vi "Add Data to EQE Log File.vi"(4 "Skip cell?":bool, 6 "Scan settings":T1={"J-V scan"=TRUE, "J-t scan"=FALSE, "Min voltage (V)"=0.0, "Max voltage (V)"=1.4, "Step (V)"=0.01, "Measurement delay (ms)"=10.0, "1st scan FB-SC"=TRUE, "Inverted structure"=FALSE, "Stabilisation time (s)"=0.0, "Stabilisation mode"=0, "Stabilisation value (V or A) "=0.0, "Step time (s)"=1.0, "Integration time"=0, "Repeat light scans"=FALSE, "Stabilisation in the dark?"=FALSE, "J-t Min (V)"=0.0, "J-t Max (V)"=1.4, "J-t Step (V)"=0.01, "Max. power stabilisation"=FALSE, "J-t 1st scan FB-SC"=TRUE, "J-t Inverted structure"=FALSE, "Max power tracking"=FALSE, "Vmp (V)"=0.7, "Total stabilisation time (s)"=100.0, "J-t best pixel only"=0, "Max power best pixel only"=0, "Vmp from J-V scan"=FALSE, "Intensity dependence"=FALSE, "P dep best pixel only"=0, "External quantum efficiency"=FALSE, "EQE best pixel only"=0, "WL min (nm)"=300.0, "WL max (nm)"=900.0, "WL step (nm)"=5.0, "Wait (ms)"=100.0, "No. of repeat scans"=2.0, "Only repeat for best pixel"=0, "Chopper Freq.  (Hz)"=90.0, "Time Constant (s)"=2.0, "Stabilisation time step (s)"=1.0, "Illumination conditions"=2, "Scan rate min (V/s)"=0.1, "Scan rate max (V/s)"=1.0, "No. of scan rate steps"=1.0, "Scan rate voltage step priority"=FALSE, "Scan rate measurement delay priority"=FALSE, "J-t Illumination conditions"=0, "White bias  (no. of suns)"=200.0, "Max P stab. Specific voltage"=FALSE} {"J-t Illumination conditions" items=["Light only", "Dark only", "Light then dark", "Dark then light"]; "No. of scan rate steps" min=1.0 step=1.0; "Illumination conditions" items=["Light only", "Dark only", "Light then dark", "Dark then light", "Light then dark then light", "Dark then light then dark"]; "Time Constant (s)" items=["0.003", "0.01", "0.03", "0.1", "0.3", "1", "3", "10", "30", "100"]; "Only repeat for best pixel" items=["only for best pixel", "for best 2 pixels", "for best 3 pixels", "for best 4 pixels", "for best 5 pixels", "for best 6 pixels", "for best 7 pixels", "for all pixels"]; "No. of repeat scans" min=1.0 step=1.0; "EQE best pixel only" items=["only the best pixel", "the best 2 pixel", "the best 3 pixel", "the best 4 pixel", "the best 5 pixel", "the best 6 pixel", "the best 7 pixel", "all pixels"]; "P dep best pixel only" items=["only the best pixel", "the best 2 pixels", "the best 3 pixels", "the best 4 pixels", "the best 5 pixels", "the best 6 pixels", "the best 7 pixels", "all pixels"]; "Max power best pixel only" items=["only the best pixel", "the best 2 pixels", "the best 3 pixels", "the best 4 pixels", "the best 5 pixels", "the best 6 pixels", "the best 7 pixels", "all pixels"]; "J-t best pixel only" items=["only the best pixel", "the best 2 pixels", "the best 3 pixels", "the best 4 pixels", "the best 5 pixels", "the best 6 pixels", "the best 7 pixels", "all pixels"]; "Integration time" items=["Fast", "Normal", "High Accuracy"]; "Stabilisation mode" items=["V", "I"]; "Measurement delay (ms)" min=10.0}, 7 "Cell details cluster":T3={"Cell Position"=16, "Cell Label"="", "Pixel to measure"=0, "Area (cm^2)"=0.126, "Variable"="", "Variable value"="", "Scan settings in queue"=0, "Light or dark"="", "Measurement Type"=""} {"Pixel to measure" items=["All", "1", "2", "3", "4", "5", "6", "7", "8"]}, 8 "EQE Data Output Folder":path, 9 "Mismatch Factor":dbl, 10 "Jsc @ 1 sun (mA/cm^2)":dbl, 11 "File path for EQE data":path) -> (0 "File path for EQE image":path, 1 "EQE Curve":cluster{"all rows":dbl[], "all rows":dbl[]}[](graph) caption="JV Curve", 2 "File path for master log":path, 3 "Master Log":string[][](table))   [LabVIEW 2011]
uses:
  TypeDefs/Scan settings.ctl
  TypeDefs/Settings Boolean.ctl
  <vilib>/Utility/file.llb/Read From Spreadsheet File (DBL).vi
  <vilib>/Utility/file.llb/Write To Spreadsheet File (string).vi
  <vilib>/Utility/file.llb/Read From Spreadsheet File (string).vi
panel:
  in  "Experiment title":string
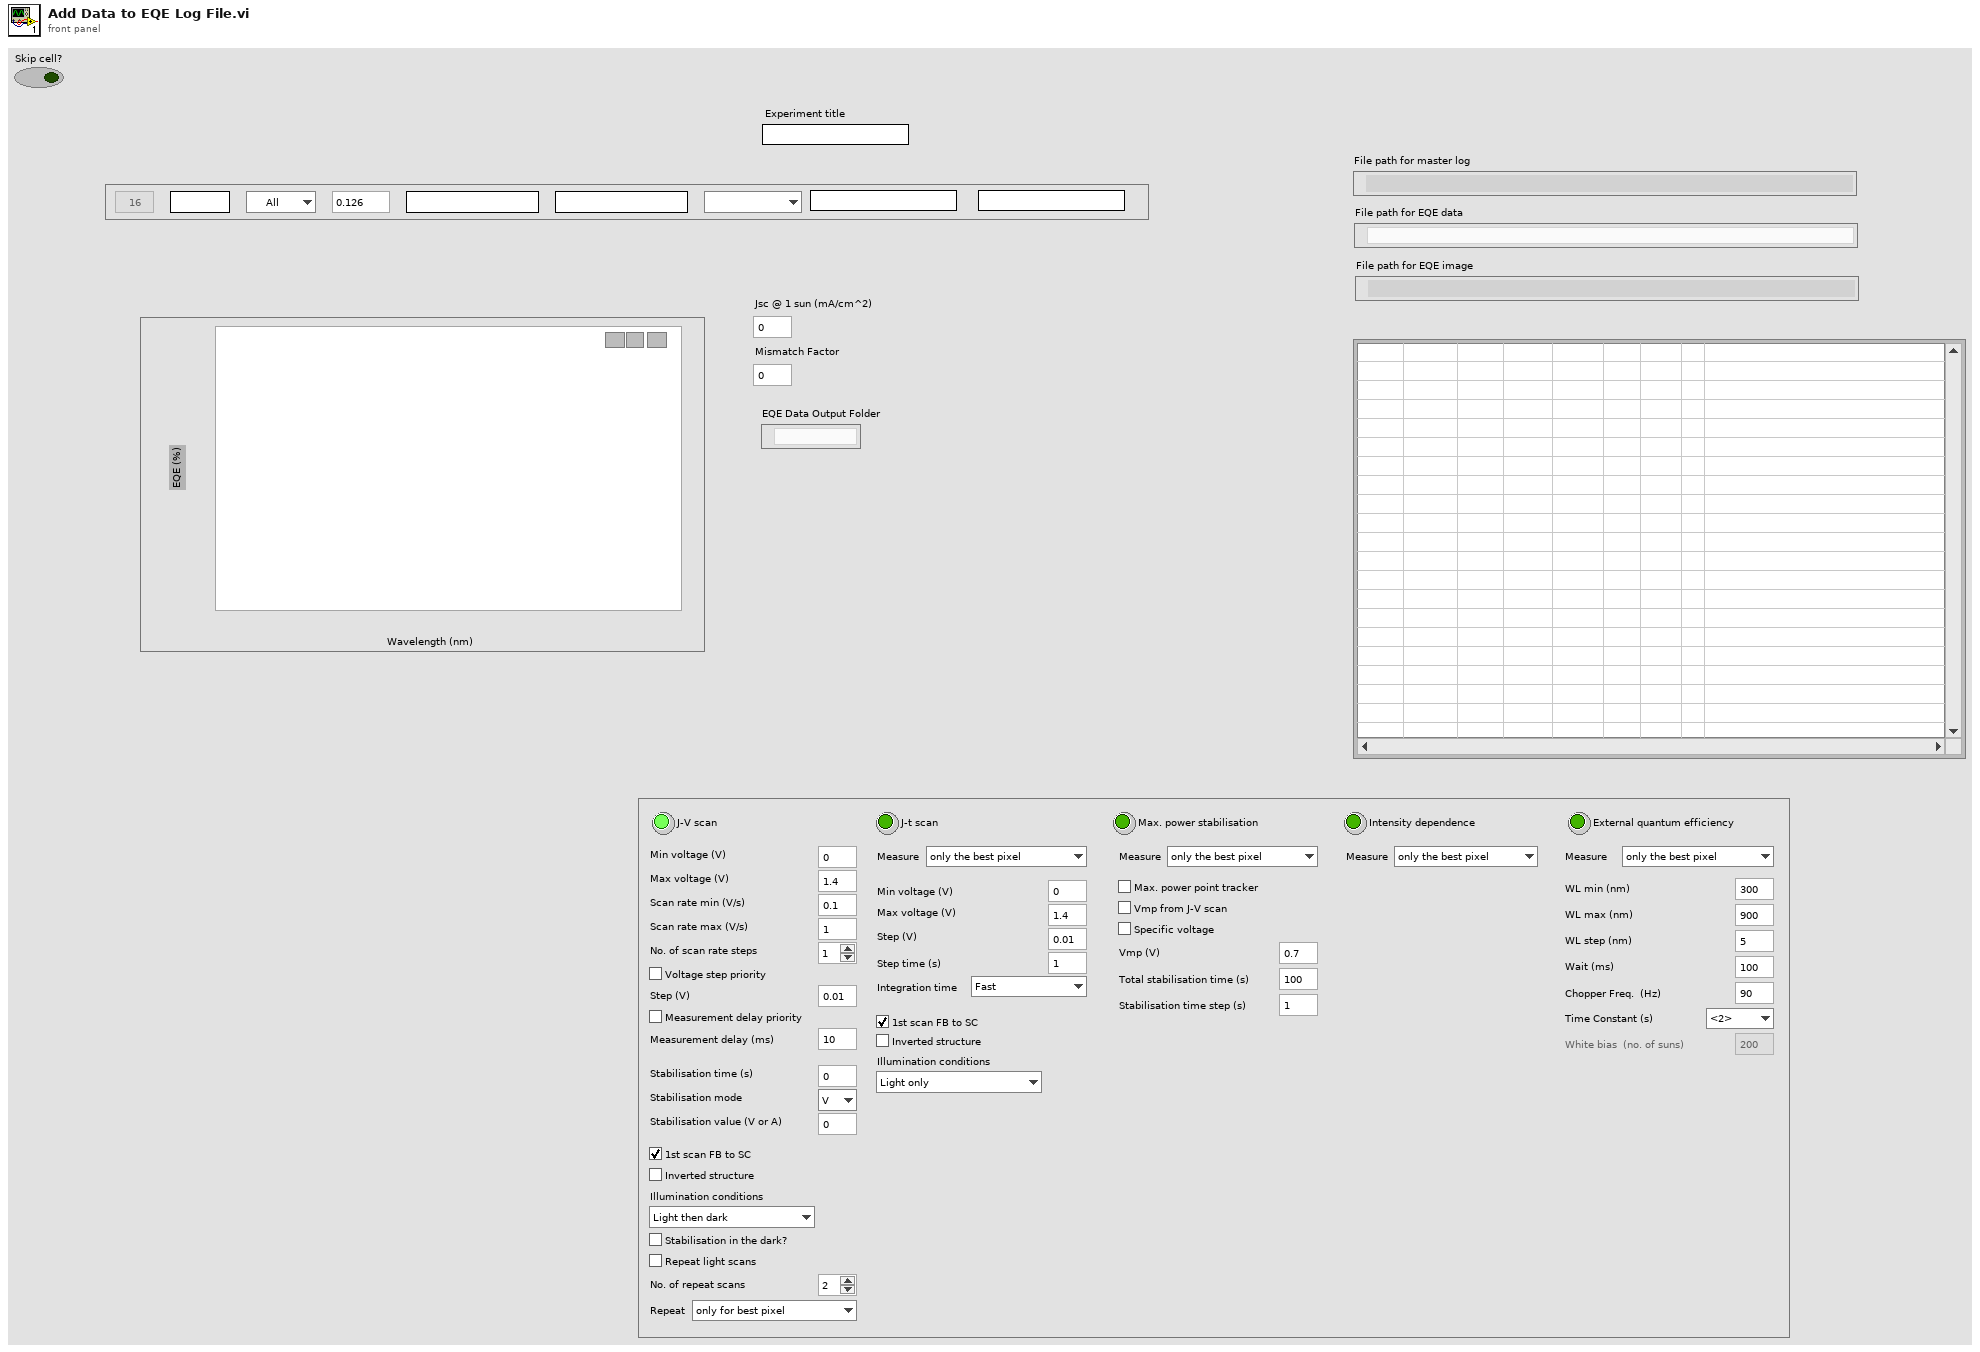
[diagram p1: front panel]
types:
  T1 = typedef "Scan settings.ctl" = cluster{"J-V scan":T2, "J-t scan":bool, "Min voltage (V)":dbl, "Max voltage (V)":dbl, "Step (V)":dbl, "Measurement delay (ms)":dbl, "1st scan FB-SC":bool, "Inverted structure":bool, "Stabilisation time (s)":dbl, "Stabilisation mode":u16, "Stabilisation value (V or A) ":dbl, "Step time (s)":dbl, "Integration time":u16, "Repeat light scans":bool, "Stabilisation in the dark?":bool, "J-t Min (V)":dbl, "J-t Max (V)":dbl, "J-t Step (V)":dbl, "Max. power stabilisation":bool, "J-t 1st scan FB-SC":bool, "J-t Inverted structure":bool, "Max power tracking":bool, "Vmp (V)":dbl, "Total stabilisation time (s)":dbl, "J-t best pixel only":u16, "Max power best pixel only":u16, "Vmp from J-V scan":bool, "Intensity dependence":bool, "P dep best pixel only":u16, "External quantum efficiency":bool, "EQE best pixel only":u16, "WL min (nm)":dbl, "WL max (nm)":dbl, "WL step (nm)":dbl, "Wait (ms)":dbl, "No. of repeat scans":dbl, "Only repeat for best pixel":u16, "Chopper Freq.  (Hz)":dbl, "Time Constant (s)":dbl, "Stabilisation time step (s)":dbl, "Illumination conditions":u16, "Scan rate min (V/s)":dbl, "Scan rate max (V/s)":dbl, "No. of scan rate steps":dbl, "Scan rate voltage step priority":bool, "Scan rate measurement delay priority":bool, "J-t Illumination conditions":u16, "White bias  (no. of suns)":dbl, "Max P stab. Specific voltage":bool}
  T2 = typedef "Settings Boolean.ctl" = bool
  T3 = cluster{"Cell Position":i32, "Cell Label":string, "Pixel to measure":u16, "Area (cm^2)":dbl, "Variable":string, "Variable value":string, "Scan settings in queue":u16, "Light or dark":string, "Measurement Type":string}
  T4 = typedef "imagedata.ctl" = cluster{"image type":i32, "image depth":i32, "image":u8[], "mask":u8[], "colors":u32[], "Rectangle":cluster{"left":i16, "top":i16, "right":i16, "bottom":i16}}
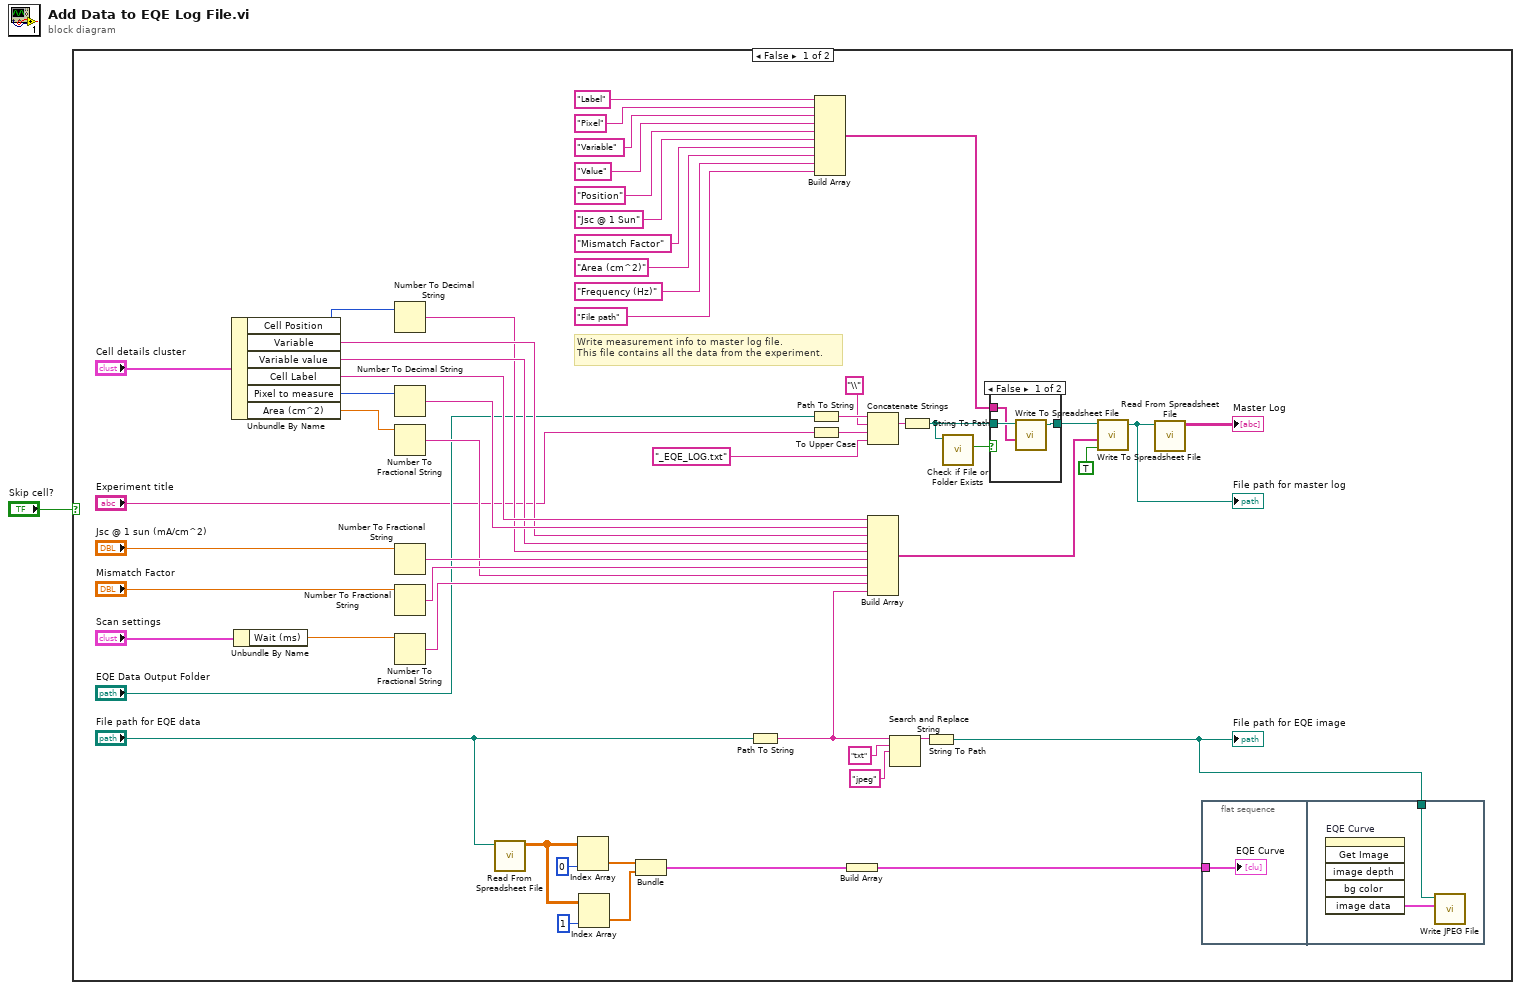
[diagram p0: block diagram]
diagram:
  n1 = case shown="False" "Skip cell?" {
    frame False {
      # "Write measurement info to master log file.\nThis file contains all the data from the experiment."
      n2 = Unbundle By Name("Cell details cluster") -> ("Cell Position"=w42:i32, "Variable"=w20:string, "Variable value"=w19:string, "Cell Label"=w41:string, "Pixel to measure"=w43:u16, "Area (cm^2)"=w24:dbl)
      n3 = Unbundle By Name("Scan settings") -> ("Wait (ms)"=w23:dbl)
      n4 = Number To Decimal String(number=w42) -> (decimal integer string=w18:string)  [unwired: 1 in]
      n5 = Number To Decimal String(number=w43) -> (decimal integer string=w40:string)  [unwired: 1 in]
      n6 = Number To Fractional String(number=w24) -> (F-format string=w15:string)  [unwired: 3 in]
      n7 = Number To Fractional String(number="Jsc @ 1 sun (mA/cm^2)") -> (F-format string=w17:string)  [unwired: 3 in]
      n8 = Number To Fractional String(number="Mismatch Factor") -> (F-format string=w16:string)  [unwired: 3 in]
      n9 = Number To Fractional String(number=w23) -> (F-format string=w14:string)  [unwired: 3 in]
      n10 = call-poly <vilib>:"Read From Spreadsheet File.vi"("file path (dialog if empty)"="File path for EQE data") -> ("all rows"=w9:dbl[][])  [unwired: 6 in, 4 out]
      n11 = Index Array(array=w9, index (col)=0 ("disabled index (col)")) -> (element=w6:dbl[])  [unwired: 1 in]
      n12 = Index Array(array=w9, index (col)=1 ("disabled index (col)")) -> (element=w5:dbl[])  [unwired: 1 in]
      n13 = Bundle("all rows"=w6, "all rows"=w5) -> (w4:cluster{"all rows":dbl[], "all rows":dbl[]})  [unwired: 1 in]
      n14 = Path To String(path="File path for EQE data") -> (string=w13:string)
      n15 = Path To String(path="EQE Data Output Folder") -> (string=w56:string)
      n16 = To Upper Case(1:"Experiment title") -> (0:w45:string)
      n17 = Build Array("Label", "Pixel", "Variable", "Value", "Position", "Jsc @ 1 Sun", "Mismatch Factor", "Area (cm^2)", "Frequency (Hz)", "File path") -> (w36:string[])
      n18 = Build Array(w4) -> (w3:cluster{"all rows":dbl[], "all rows":dbl[]}[])
      n19 = Concatenate Strings(w56, "\\", w45, "_EQE_LOG.txt") -> (w54:string)
      n20 = Build Array(w41, w40, w20, w19, w18, w17, w16, w15, w14, w13) -> (w53:string[])
      n21 = Search and Replace String(input string=w13, search string="txt", replace string="jpeg") -> (result string=w50:string)  [unwired: 5 in, 3 out]
      n22 = String To Path(string=w54) -> (path=w38:path)
      n23 = String To Path(string=w50) -> (path=w2:path)
      "File path for EQE image" <- w2
      n24 = call <vilib>:"Check if File or Folder Exists.vi"("path"=w38) -> ("file or folder exists?"=w39:bool)  [unwired: 8 in, 2 out]
      n25 = case shown="False" w39 {
        tunnel: w38 -> [w62 w63]
        tunnel: [w61 w63] -> w37
        tunnel: w36 -> [w60 _]
        frame False {
          n26 = call-poly <vilib>:"Write To Spreadsheet File.vi"("1D data"=w60, "file path (dialog if empty)"=w62) -> ("new file path (Not A Path if cancelled)"=w61:path)  [unwired: 6 in]
        }
        frame True {
        }
      }
      n27 = call-poly <vilib>:"Write To Spreadsheet File.vi"("append to file? (new file:F)"=TRUE, "1D data"=w53, "file path (dialog if empty)"=w37) -> ("new file path (Not A Path if cancelled)"=w48:path)  [unwired: 5 in]
      "File path for master log" <- w48
      n28 = call-poly <vilib>:"Read From Spreadsheet File.vi"("file path (dialog if empty)"=w48) -> ("all rows"=→"Master Log":string[][])  [unwired: 6 in, 4 out]
      n29 = flat-sequence {
        tunnel: w3 -> [w57]
        tunnel: w2 -> [w58]
        frame #0 {
          "EQE Curve" <- w57
        }
        frame #1 {
          n30 = invoke on="EQE Curve" class="XYGraph (strict)" method="Get Image"() -> ("image data"=w59:T4)  [unwired: 6 in, 5 out]
          n31 = call <vilib>:"Write JPEG File.vi"("image data"=w59, "path to JPEG file"=w58) -> ()  [unwired: 8 in, 2 out]
        }
      }
    }
    frame True {
    }
  }
